vi "Configure Voltage High Limit.vi"(0 "VISA resource name":refnum<visa-resource-name>, 5 "Voltage High Limit (300 V)":dbl=300.0 min=0.0 max=400.0 format="%.1f", 11 "error in (no error)":errorcluster) -> (4 "VISA resource name out":refnum<visa-resource-name>, 15 "error out":errorcluster)   [LabVIEW 2020, in "eec 6700.lvlib"]
doc: "Set the <B>voltage high limit</B> in the power source instrument.\n\n<B>Range</B>\n<B>For AC</B>: 0.0~300.0 V\n\nThe Voltage High-Limit configures a maximum voltage threshold or ceiling level when programming the output voltage in the testing parameters screen.\nIf the output voltage is above the ceiling level, the instrument will fail the test"
uses:
  <instrlib>/eec 6700/eec 6700.lvlib
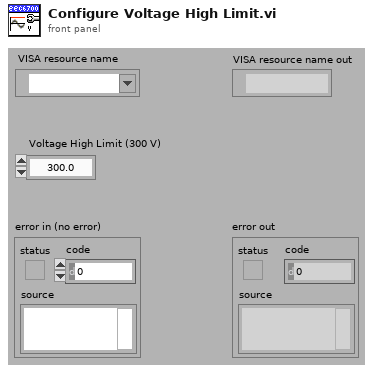
[diagram p1: front panel]
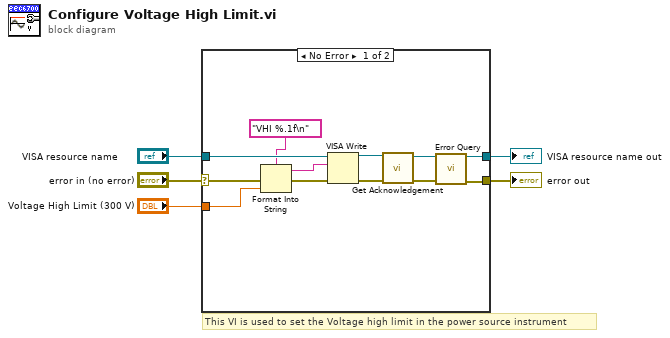
[diagram p0: block diagram]
diagram:
  # "This VI is used to set the Voltage high limit in the power source instrument"
  n1 = case shown="No Error" "error in (no error)" {
    selector: "error in (no error)" -> [w11 w19]
    tunnel: [w12 w19] -> w5
    tunnel: [w13 w18] -> w4
    tunnel: "VISA resource name" -> [w17 w18]
    tunnel: "Voltage High Limit (300 V)" -> [w16 _]
    frame No Error {
      n2 = Format Into String(format string="VHI %.1f\n" ("Command"), error in=w11, w16) -> (resulting string=w15:string, error out=w10:errorcluster)  [unwired: 1 in]
      n3 = VISA Write(VISA resource name=w17, write buffer=w15, error in (no error)=w10) -> (VISA resource name out=w6:refnum<visa-resource-name>, error out=w9:errorcluster)  [unwired: 1 out]
      n4 = call <instrlib>:"Get Acknowledgement.vi"("VISA resource name"=w6, "error in (no error)"=w9) -> ("VISA resource name out"=w7:refnum<visa-resource-name>, "error out"=w8:errorcluster)  [unwired: 12 in]
      n5 = call <instrlib>:"Error Query.vi"("VISA resource name"=w7, "error in (no error)"=w8) -> ("VISA resource name out"=w13:refnum<visa-resource-name>, "error out"=w12:errorcluster)  [unwired: 10 in, 2 out]
    }
    frame Error {
    }
  }
  "error out" <- w5
  "VISA resource name out" <- w4
